vi "ini_object_load.vi"(7 "generate error if unsuppoted data type (true)":bool=TRUE, 8 "error in":errorcluster, 10 "auto ini row":T1, 11 "refnum in":T2) -> (0 "error out":errorcluster, 3 "refnum out":T2)   [LabVIEW 2013]
uses:
  <vilib>/Utility/config.llb/Config Data RefNum.ctl
  ini_parse_row.ctl
  <vilib>/Utility/config.llb/Read Key (String).vi
  <vilib>/regexp/Match Regular Expression.xnode
  <vilib>/Utility/config.llb/NI_LVConfig.lvlib
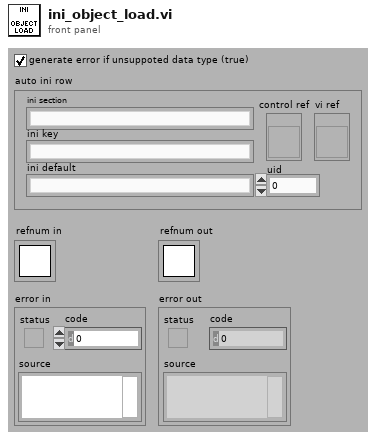
[diagram p1: front panel]
types:
  T1 = typedef "ini_parse_row.ctl" = cluster{"ini section":string, "ini key":string, "ini default":string, "control ref":refnum<vi>, "uid":i32, "vi ref":refnum<vi>}
  T2 = typedef "NI_LVConfig.lvlib/Config Data RefNum.ctl" = refnum<k1>
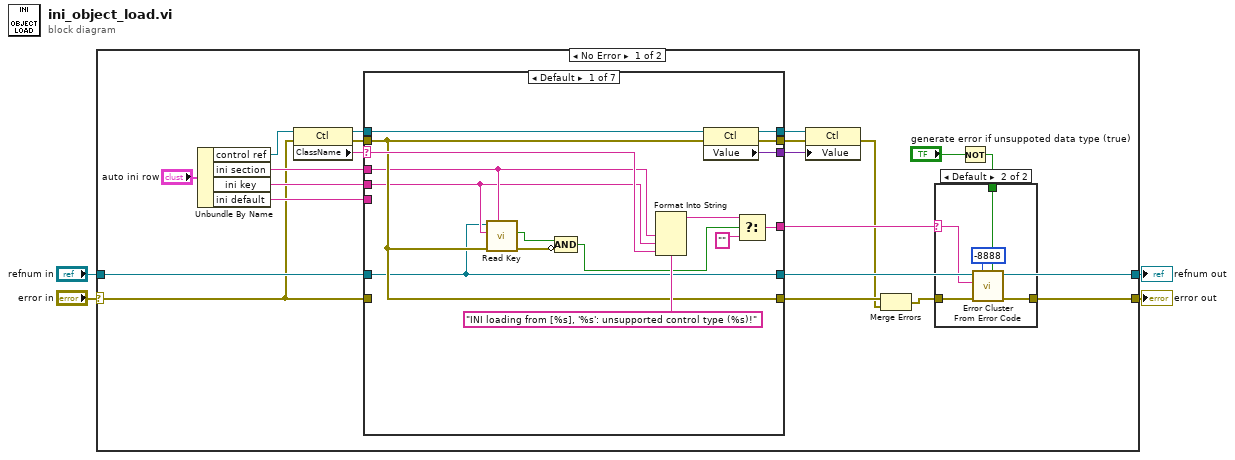
[diagram p0: block diagram]
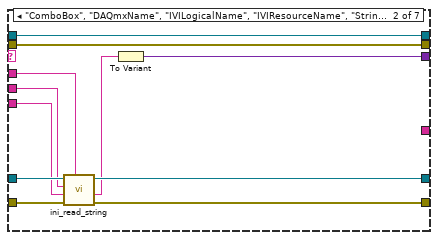
[diagram p3: hidden frame]
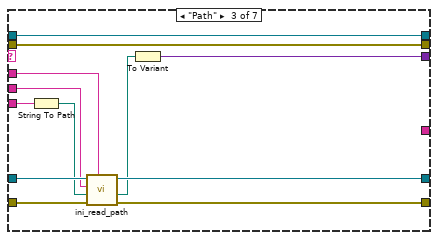
[diagram p4: hidden frame]
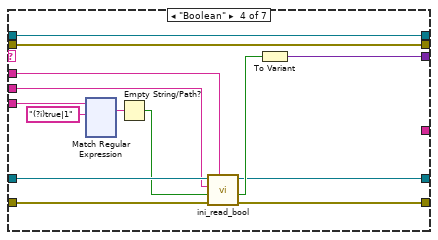
[diagram p5: hidden frame]
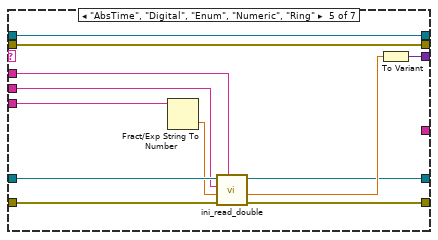
[diagram p6: hidden frame]
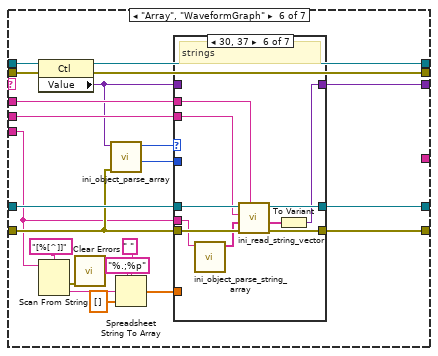
[diagram p7: hidden frame]
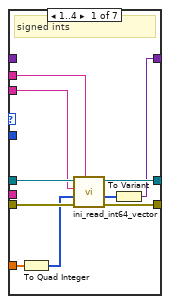
[diagram p8: hidden frame]
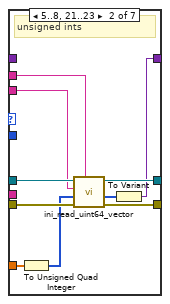
[diagram p9: hidden frame]
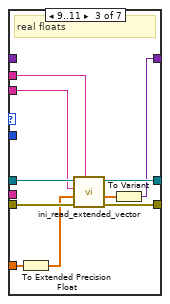
[diagram p10: hidden frame]
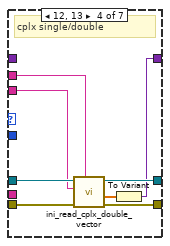
[diagram p11: hidden frame]
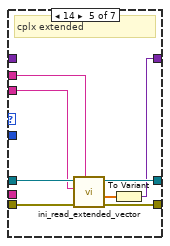
[diagram p12: hidden frame]
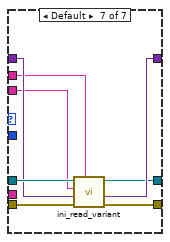
[diagram p13: hidden frame]
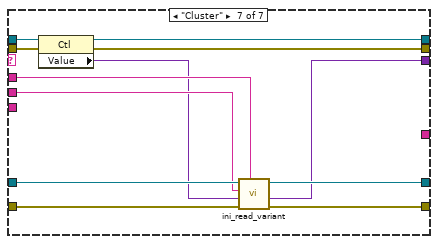
[diagram p14: hidden frame]
diagram:
  n1 = case shown="No Error" "error in" {
    selector: "error in" -> [w5 w310]
    tunnel: "refnum in" -> [w25 w309]
    tunnel: [w24 w309] -> w3
    tunnel: [w15 w310] -> w2
    frame No Error {
      n2 = Unbundle By Name("auto ini row") -> ("control ref"=w20:refnum<vi>, "ini section"=w22:string, "ini key"=w21:string, "ini default"=w18:string)
      n3 = property class="Ctl"(reference=w20, error in=w5) -> (reference out=w16:refnum<vi>, error out=w17:errorcluster, "ClassName"=w19:string)
      n4 = case shown="Default" w19 {
        selector: w19 -> [w46 _ _ _ _ _ _]
        tunnel: [w39 w55 w67 w74 w202 w229 w305] -> w8
        tunnel: w25 -> [w32 w57 w69 w82 w209 w232 w308]
        tunnel: [w32 w56 w68 w73 w201 w228 w304] -> w24
        tunnel: w22 -> [w34 w54 w66 w81 w208 w231 w307]
        tunnel: w21 -> [w33 w53 w65 w80 w207 w230 w306]
        tunnel: w18 -> [_ w52 w64 w78 w206 w211 _]
        tunnel: w17 -> [w39 w49 w61 w72 w200 w220 w303]
        tunnel: w16 -> [w42 w48 w60 w71 w199 w219 w302]
        tunnel: [w38 _ _ _ _ _ _] -> w14
        tunnel: w5 -> [_ w58 w70 w83 w210 w216 w299]
        tunnel: [w43 w50 w62 w79 w204 w213 w297] -> w11
        tunnel: [w44 w49 w61 w72 w200 w218 w301] -> w10
        tunnel: [w45 w48 w60 w71 w199 w217 w300] -> w9
        frame Default {
          n5 = call-poly <vilib>:"Read Key.vi"("section"=w34, "error in (no error)"=w39, "key"=w33, "refnum"=w32) -> ("error out"=w40:errorcluster, "found?"=w41:bool)  [unwired: 4 in, 2 out]
          n6 = Compound Arithmetic op=AND(w41, invert w40) -> (w37:bool)
          n7 = Format Into String(format string="INI loading from [%s], '%s': unsupported control type (%s)!", w34, w33, w46) -> (resulting string=w36:string)  [unwired: 2 in, 1 out]
          n8 = property class="Ctl"(reference=w42, error in=w39) -> (reference out=w45:refnum<vi>, error out=w44:errorcluster, "Value"=w43:variant)
          n9 = Select(t=w36, s=w37, f="") -> (s? t:f=w38:string)
        }
        frame "ComboBox", "DAQmxName", "IVILogicalName", "IVIResourceName", "String", "VISAResourceName" {
          n10 = call "ini_read_string.vi"("section"=w54, "error in"=w58, "default value"=w52, "key"=w53, "refnum in"=w57) -> ("error out"=w55:errorcluster, "value"=w51:string, "refnum out"=w56:T2)  [unwired: 3 in, 1 out]
          n11 = To Variant(anything=w51) -> (Variant=w50:variant)
        }
        frame "Path" {
          n12 = String To Path(string=w64) -> (path=w59:path)
          n13 = call "ini_read_path.vi"("section"=w66, "error in"=w70, "default value"=w59, "key"=w65, "refnum in"=w69) -> ("error out"=w67:errorcluster, "value"=w63:path, "refnum out"=w68:T2)  [unwired: 3 in, 1 out]
          n14 = To Variant(anything=w63) -> (Variant=w62:variant)
        }
        frame "Boolean" {
          n15 = xnode "Match Regular Expression"("input string"=w78, "regular expression"="(?i)true|1") -> ("whole match"=w76:string)  [unwired: 4 in, 4 out]
          n16 = Empty String/Path?(string/path=w76) -> (empty?=w75:bool)
          n17 = call "ini_read_bool.vi"("section"=w81, "error in"=w83, "default value"=w75, "key"=w80, "refnum in"=w82) -> ("error out"=w74:errorcluster, "value"=w84:bool, "refnum out"=w73:T2)  [unwired: 3 in, 1 out]
          n18 = To Variant(anything=w84) -> (Variant=w79:variant)
        }
        frame "AbsTime", "Digital", "Enum", "Numeric", "Ring" {
          n19 = Fract/Exp String To Number(string=w206) -> (number=w205:dbl)  [unwired: 3 in, 1 out]
          n20 = call "ini_read_double.vi"("section"=w208, "error in"=w210, "default value"=w205, "key"=w207, "refnum in"=w209) -> ("error out"=w202:errorcluster, "value"=w203:dbl, "refnum out"=w201:T2)  [unwired: 3 in, 1 out]
          n21 = To Variant(anything=w203) -> (Variant=w204:variant)
        }
        frame "Array", "WaveformGraph" {
          n22 = property class="Ctl"(reference=w219, error in=w220) -> (reference out=w217:refnum<vi>, error out=w218:errorcluster, "Value"=w214:variant)
          n23 = Scan From String(format string="[%[^]]", input string=w211) -> (error out=w222:errorcluster, output 1=w226:string)  [unwired: 3 in, 2 out]
          n24 = call <vilib>:"Clear Errors.vi"("error in (no error)"=w222) -> ()  [unwired: 6 in, 1 out]
          n25 = call "ini_object_parse_array.vi"("error in"=w216, "variant in"=w214) -> ("dims"=w212:i16, "type id"=w215:i16)  [unwired: 6 in, 2 out]
          n26 = Spreadsheet String To Array(delimiter (Tab)=" ", format string="%.;%p", spreadsheet string=w226, array type (2D Dbl)=ext[] []) -> (array=w221:ext[])
          n27 = case shown="30, 37" w215 {
            tunnel: w232 -> [w242 w252 w262 w270 w278 w288 w292]
            tunnel: w231 -> [w241 w251 w261 w269 w277 w287 w290]
            tunnel: w230 -> [w240 w250 w260 w268 w276 w286 w289]
            tunnel: [w235 w245 w255 w264 w272 w282 w295] -> w213
            tunnel: [w239 w249 w259 w267 w275 w285 w294] -> w229
            tunnel: [w238 w248 w258 w266 w274 w284 w293] -> w228
            tunnel: w221 -> [w237 w247 w257 _ _ _ _]
            tunnel: w216 -> [w236 w246 w256 w265 w273 w283 w296]
            tunnel: w214 -> [_ _ _ _ _ _ w291]
            tunnel: w212 -> [_ _ _ _ _ _ _]
            tunnel: w211 -> [_ _ _ _ _ w279 _]
            frame 1..4 {
              # "signed ints"
              n28 = To Quad Integer(1:w237) -> (0:w233:i64[])
              n29 = call "ini_read_int64_vector.vi"("section"=w241, "error in"=w236, "default"=w233, "key"=w240, "refnum in"=w242) -> ("error out"=w239:errorcluster, "values"=w234:i64[], "refnum out"=w238:T2)  [unwired: 3 in, 1 out]
              n30 = To Variant(anything=w234) -> (Variant=w235:variant)
            }
            frame 5..8, 21..23 {
              # "unsigned ints"
              n31 = To Unsigned Quad Integer(1:w247) -> (0:w243:u64[])
              n32 = call "ini_read_uint64_vector.vi"("section"=w251, "error in"=w246, "default"=w243, "key"=w250, "refnum in"=w252) -> ("error out"=w249:errorcluster, "values"=w244:u64[], "refnum out"=w248:T2)  [unwired: 3 in, 1 out]
              n33 = To Variant(anything=w244) -> (Variant=w245:variant)
            }
            frame 9..11 {
              # "real floats"
              n34 = To Extended Precision Float(1:w257) -> (0:w253:ext[])
              n35 = call "ini_read_extended_vector.vi"("section"=w261, "error in"=w256, "default"=w253, "key"=w260, "refnum in"=w262) -> ("error out"=w259:errorcluster, "values"=w254:ext[], "refnum out"=w258:T2)  [unwired: 3 in, 1 out]
              n36 = To Variant(anything=w254) -> (Variant=w255:variant)
            }
            frame 12, 13 {
              # "cplx single/double"
              n37 = call "ini_read_cplx_double_vector.vi"("section"=w269, "error in"=w265, "key"=w268, "refnum in"=w270) -> ("error out"=w267:errorcluster, "values"=w263:cdb[], "refnum out"=w266:T2)  [unwired: 4 in, 1 out]
              n38 = To Variant(anything=w263) -> (Variant=w264:variant)
            }
            frame 14 {
              # "cplx extended"
              n39 = call "ini_read_extended_vector.vi"("section"=w277, "error in"=w273, "key"=w276, "refnum in"=w278) -> ("error out"=w275:errorcluster, "values"=w271:ext[], "refnum out"=w274:T2)  [unwired: 4 in, 1 out]
              n40 = To Variant(anything=w271) -> (Variant=w272:variant)
            }
            frame 48, 55 {
              # "strings"
              n41 = call "ini_object_parse_string_array.vi"("string in"=w279) -> ("string array out"=w280:string[])  [unwired: 9 in, 1 out]
              n42 = call "ini_read_string_vector.vi"("section"=w287, "error in"=w283, "default"=w280, "key"=w286, "refnum in"=w288) -> ("error out"=w285:errorcluster, "values"=w281:string[], "refnum out"=w284:T2)  [unwired: 3 in, 1 out]
              n43 = To Variant(anything=w281) -> (Variant=w282:variant)
            }
            frame Default {
              n44 = call "ini_read_variant.vi"("section"=w290, "error in"=w296, "default"=w291, "key"=w289, "refnum in"=w292) -> ("error out"=w294:errorcluster, "variant out"=w295:variant, "refnum out"=w293:T2)  [unwired: 3 in, 1 out]
            }
          }
        }
        frame "Cluster" {
          n45 = property class="Ctl"(reference=w302, error in=w303) -> (reference out=w300:refnum<vi>, error out=w301:errorcluster, "Value"=w298:variant)
          n46 = call "ini_read_variant.vi"("section"=w307, "error in"=w299, "default"=w298, "key"=w306, "refnum in"=w308) -> ("error out"=w305:errorcluster, "variant out"=w297:variant, "refnum out"=w304:T2)  [unwired: 3 in, 1 out]
        }
      }
      n47 = property class="Ctl"(reference=w9, error in=w10, "Value"=w11) -> (error out=w7:errorcluster)  [unwired: 1 out]
      n48 = Merge Errors(w8, w7) -> (w6:errorcluster)
      n49 = Not(x="generate error if unsuppoted data type (true)") -> (.not. x?=w12:bool)
      n50 = case shown="Default" w14 {
        selector: w14 -> [_ w28]
        tunnel: w6 -> [w26 w31]
        tunnel: [w26 w30] -> w15
        tunnel: w12 -> [_ w27]
        frame "" {
        }
        frame Default {
          n51 = call <vilib>:"Error Cluster From Error Code.vi"("is warning? (False)"=w27, "error in (no error)"=w31, "error message (\"\")"=w28, "error code (0)"=-8888) -> ("error out"=w30:errorcluster)  [unwired: 5 in]
        }
      }
    }
    frame Error {
    }
  }
  "error out" <- w2
  "refnum out" <- w3
